vi "Hardware ports Config.vi"(9 "Ring Refnum":refnum<vi>, 11 "Configuration Folder path":path) -> (2 "data":T1(array[cluster]))   [LabVIEW 2020]
uses:
  <vilib>/Instr/_visa.llb/VISA Configure Serial Port (Instr).vi
panel:
  out "error out":errorcluster
  in  "error in (no error)":errorcluster
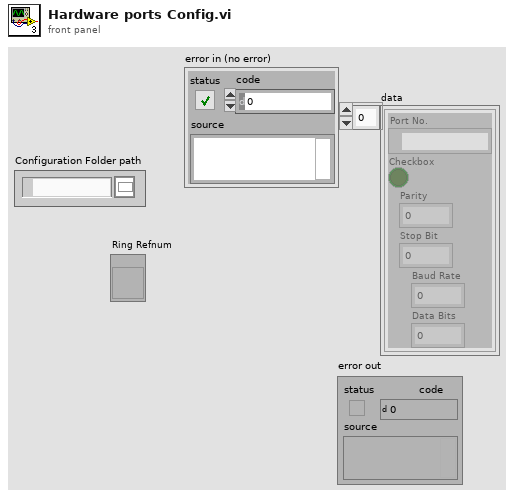
[diagram p1: front panel]
types:
  T1 = cluster{"Port No.":refnum<visa-resource-name>, "Checkbox":bool, "Parity":u16, "Stop Bit":u16, "Baud Rate":u32, "Data Bits":u8}[]
  T2 = typedef "Port details.ctl" = cluster{"Port No.":refnum<visa-resource-name>, "Checkbox":bool, "Parity":u16, "Stop Bit":u16, "Baud Rate":u32, "Data Bits":u8}
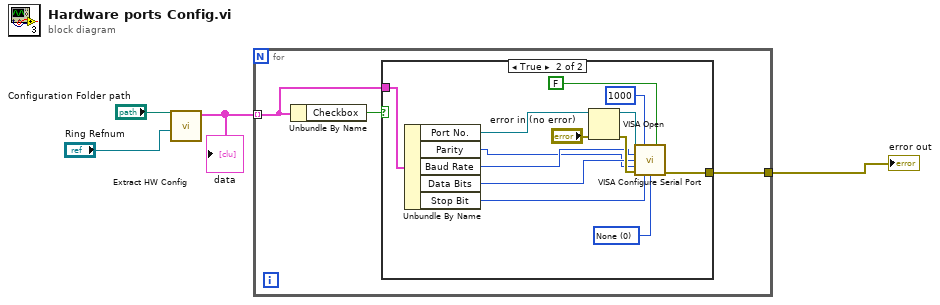
[diagram p0: block diagram]
diagram:
  n1 = call "Extract HW Config.vi"("Ring Refnum"="Ring Refnum", "Configuration Folder Path"="Configuration Folder path") -> ("Channel 2"=w4:T2[])  [unwired: 9 in]
  "data" <- w4
  n2 = for {
    tunnel: w4 -> [w6] mode=indexing
    tunnel: [w5] -> w1
    n3 = Unbundle By Name(w6) -> ("Checkbox"=w7:bool)
    n4 = case shown="True" w7 {
      tunnel: w6 -> [_ w18]
      tunnel: [_ w8] -> w5
      frame False {
      }
      frame True {
        w10 = u16 0 items=["None", "XON/XOFF", "RTS/CTS", "XON/XOFF & RTS/CTS", "DTR/DSR", "XON/XOFF & DTR/DSR"] ("flow control (0:none)")
        n5 = Unbundle By Name(w18) -> ("Port No."=w15:refnum<visa-resource-name>, "Parity"=w14:u16, "Baud Rate"=w17:u32, "Data Bits"=w16:u8, "Stop Bit"=w11:u16)
        n6 = VISA Open(error in (no error)="error in (no error)", VISA resource name=w15) -> (VISA resource name=w20:refnum<visa-resource-name>, error out=w19:errorcluster)  [unwired: 3 in]
        n7 = call-poly "VISA Configure Serial Port"("VISA resource name"=w20, "timeout (10sec)"=u32 1000, "Enable Termination\nChar (T)"=FALSE ("Enable Termination\nChar (T)"), "baud rate (9600)"=w17, "data bits (8)"=w16, "parity (0:none)"=w14, "error in (no error)"=w19, "stop bits (10: 1 bit)"=w11, "flow control (0:none)"=w10) -> ("error out"=w8:errorcluster)  [unwired: 5 in, 1 out]
      }
    }
  }
  "error out" <- w1
